vi "Main RT CK.vi"() -> ()   [LabVIEW 2020]
uses:
  Shared/Control/State - eFGV.ctl
  Control/MQTT Send Data.ctl
panel:
  in  "stop":bool
  out "error in (no error) 2":errorcluster
  in  "error in (no error)":errorcluster
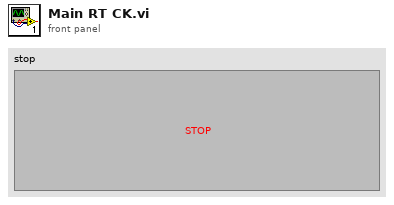
[diagram p1: front panel]
types:
  T1 = typedef "State - eFGV.ctl" = enum16{"Init", "Read", "Write", "Close"}
  T2 = typedef "MQTT Send Data.ctl" = cluster{"Sender Module":string, "Receiving Module":string, "Topic":string, "Data":variant}
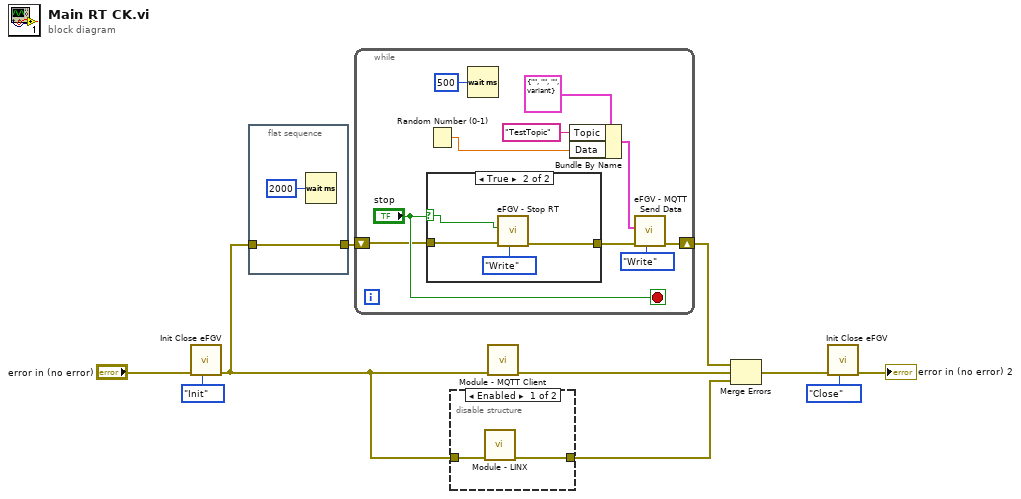
[diagram p0: block diagram]
diagram:
  n1 = call "Init Close eFGV.vi"("State"=State_-_eFGV."Init", "error in (no error)"="error in (no error)") -> ("error out"=w2:errorcluster)  [unwired: 9 in]
  n2 = flat-sequence {
    tunnel: w2 -> [w12]
    tunnel: [w12] -> w1
    frame #0 {
      n3 = Wait (ms)(milliseconds to wait=u32 2000) -> ()  [unwired: 1 out]
    }
  }
  n4 = while {
    shift-right: [w18] -> w4
    shift-left: w1 -> [w20]
    stop <- "stop" stop-if-true
    n5 = Random Number (0-1)() -> (number: 0 to 1=w14:dbl)
    n6 = case shown="True" "stop" {
      selector: "stop" -> [_ w25]
      tunnel: w20 -> [w23 w27]
      tunnel: [w23 w24] -> w19
      frame False {
      }
      frame True {
        n7 = call "eFGV - Stop RT.vi"("State"=State_-_eFGV."Write", "error in (no error)"=w27, "Stop RT"=w25) -> ("error out"=w24:errorcluster)  [unwired: 7 in, 1 out]
      }
    }
    n8 = Wait (ms)(milliseconds to wait=u32 500) -> ()  [unwired: 1 out]
    n9 = Bundle By Name(cluster=T2 {"Sender Module"="", "Receiving Module"="", "Topic"="", "Data"=variant} ("MQTT Send Data"), "Topic"="TestTopic", "Data"=w14) -> (w13:T2)
    n10 = call "eFGV - MQTT Send Data.vi"("State"=State_-_eFGV."Write", "error in (no error)"=w19, "MQTT Send Data"=w13) -> ("error out"=w18:errorcluster)  [unwired: 7 in, 1 out]
  }
  n11 = disable-structure shown="Enabled" {
    disable-tunnel: w2 -> [w29 w30]
    disable-tunnel: [w28 w30] -> w3
    frame Enabled {
      n12 = call "Module - LINX.vi"("error in (no error)"=w29) -> ("error out"=w28:errorcluster)  [unwired: 10 in]
    }
    frame Disabled {
    }
  }
  n13 = call "Module - MQTT Client.vi"("error in (no error)"=w2) -> ("error in (no error) 2"=w6:errorcluster)  [unwired: 10 in]
  n14 = Merge Errors(w4, w6, w3) -> (w7:errorcluster)
  n15 = call "Init Close eFGV.vi"("State"=State_-_eFGV."Close", "error in (no error)"=w7) -> ("error out"=→"error in (no error) 2":errorcluster)  [unwired: 9 in]
